vi "Task Start.vi"(8 "error in (no error)":errorcluster, 11 "DaqControl in":refnum<class "DaqControl.lvclass">) -> (0 "error out":errorcluster, 3 "DaqControl out":refnum<class "DaqControl.lvclass">)   [LabVIEW 2020, in "VolatusDaq.lvlib" / "DaqControl.lvclass"]
uses:
  DaqControl.lvclass
  DaqControl.lvclass/DaqControl.ctl
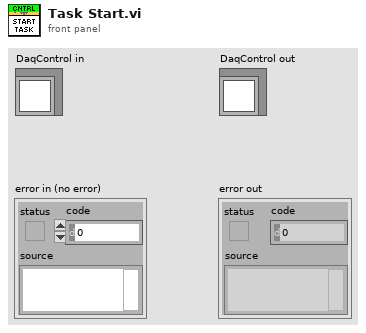
[diagram p1: front panel]
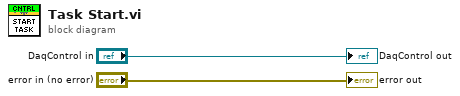
[diagram p0: block diagram]
diagram:
  "error out" <- "error in (no error)"
  "DaqControl out" <- "DaqControl in"
